vi "calcualte_jv_metrics.vi"(6 "intensity (no. of suns)":string, 9 "Data Array":dbl[][](array[numeric]), 10 "Scan settings":T2={"J-V scan"=TRUE, "Start voltage (V)"=0.0, "End voltage (V)"=0.0, "Step voltage (V)"=1.4, "Scan both directions"=TRUE, "Inverted device structure"=FALSE, "Measurement delay (ms)"=10.0, "Measurement speed"=0, "Scan rate (V/s)"=0.0, "Stabilisation time (s)"=0.0, "Stabilisation mode"=0, "Stabilisation value (V or A) "=1.0, "Illumination"=0, "Stabilisation in the dark?"=FALSE, "Repeat light scans"=FALSE, "No. of repeat scans"=0.0, "Only repeat for best pixel"=1, "J-t scan"=FALSE, "J-t best pixel only"=7, "J-t start voltage (V)"=0.0, "J-t end voltage (V)"=1.4, "J-t step voltage (V)"=0.01, "Step time (s)"=0.7, "J-t scan both directions"=TRUE, "J-t inverted device structure"=FALSE, "Settling delay (s)"=0.0, "J-t measurement speed"=0, "J-t illumination"=2, "Max. power stabilisation"=FALSE, "Max power best pixel only"=1, "Max. power point tracker"=FALSE, "Vmp from J-V scan"=FALSE, "Max P stab. Specific voltage"=FALSE, "Vmp (V)"=1.0, "Stabilisation time step (s)"=1.0, "Total stabilisation time (s)"=100.0} {"Settling delay (s)" min=0.0; "J-t illumination" items=["Light only", "Dark only", "Light then dark", "Dark then light"]; "Measurement speed" items=["Fast", "Normal", "High accuracy"]; "Illumination" items=["Light only", "Dark only", "Light then dark", "Dark then light"]; "Only repeat for best pixel" items=["only for best pixel", "for best 2 pixels", "for best 3 pixels", "for best 4 pixels", "for best 5 pixels", "for best 6 pixels", "for best 7 pixels", "for all pixels"]; "No. of repeat scans" min=1.0 step=1.0; "Max power best pixel only" items=["only the best pixel", "the best 2 pixels", "the best 3 pixels", "the best 4 pixels", "the best 5 pixels", "the best 6 pixels", "the best 7 pixels", "all pixels"]; "J-t best pixel only" items=["only the best pixel", "the best 2 pixels", "the best 3 pixels", "the best 4 pixels", "the best 5 pixels", "the best 6 pixels", "the best 7 pixels", "all pixels"]; "J-t measurement speed" items=["Fast", "Normal", "High Accuracy"]; "Stabilisation mode" items=["V", "I"]; "Measurement delay (ms)" min=10.0}, 11 "Cell details cluster":T1={"Cell Position"=16, "Cell Label"="", "Pixel to measure"=0, "Area (cm^2)"=0.126, "Variable"="", "Variable value"="", "Scan settings in queue"=0, "Light or dark"="", "Measurement type"=""} {"Pixel to measure" items=["All", "1", "2", "3", "4", "5", "6", "7", "8"]}) -> (1 "j-v metrics":string[](array[string]), 2 "j-v data":string[][](array[string]))   [LabVIEW 2016]
uses:
  TypeDefs/scan_settings.ctl
  <vilib>/Analysis/NI_AALPro.lvlib
panel:
  out "Vmp":dbl
  out "PCE":dbl
  out "FF":dbl
  out "Voc":dbl
  out "Jsc":dbl
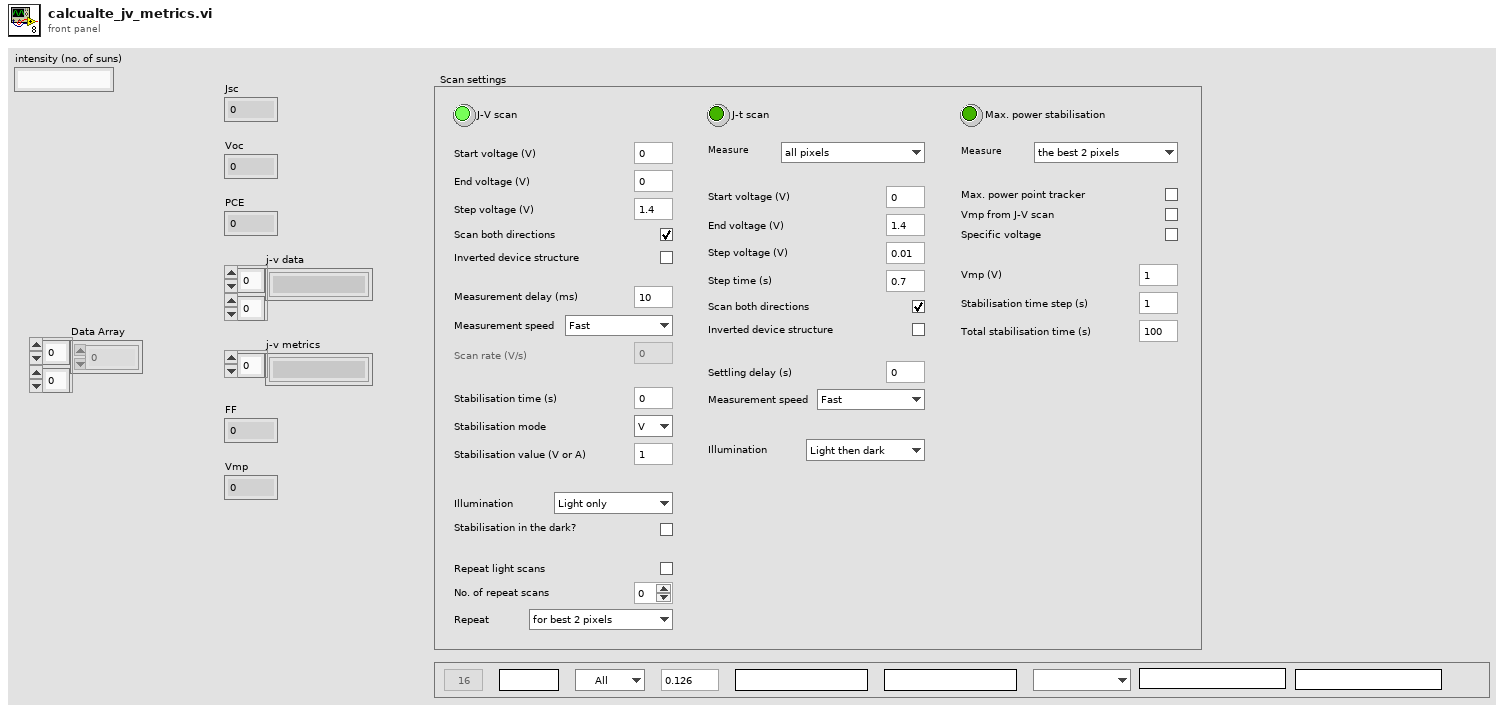
[diagram p1: front panel]
types:
  T1 = cluster{"Cell Position":i32, "Cell Label":string, "Pixel to measure":u16, "Area (cm^2)":dbl, "Variable":string, "Variable value":string, "Scan settings in queue":u16, "Light or dark":string, "Measurement type":string}
  T2 = typedef "scan_settings.ctl" = cluster{"J-V scan":bool, "Start voltage (V)":dbl, "End voltage (V)":dbl, "Step voltage (V)":dbl, "Scan both directions":bool, "Inverted device structure":bool, "Measurement delay (ms)":dbl, "Measurement speed":u8, "Scan rate (V/s)":dbl, "Stabilisation time (s)":dbl, "Stabilisation mode":u16, "Stabilisation value (V or A) ":dbl, "Illumination":u16, "Stabilisation in the dark?":bool, "Repeat light scans":bool, "No. of repeat scans":dbl, "Only repeat for best pixel":u16, "J-t scan":bool, "J-t best pixel only":u16, "J-t start voltage (V)":dbl, "J-t end voltage (V)":dbl, "J-t step voltage (V)":dbl, "Step time (s)":dbl, "J-t scan both directions":bool, "J-t inverted device structure":bool, "Settling delay (s)":dbl, "J-t measurement speed":u16, "J-t illumination":u16, "Max. power stabilisation":bool, "Max power best pixel only":u16, "Max. power point tracker":bool, "Vmp from J-V scan":bool, "Max P stab. Specific voltage":bool, "Vmp (V)":dbl, "Stabilisation time step (s)":dbl, "Total stabilisation time (s)":dbl}
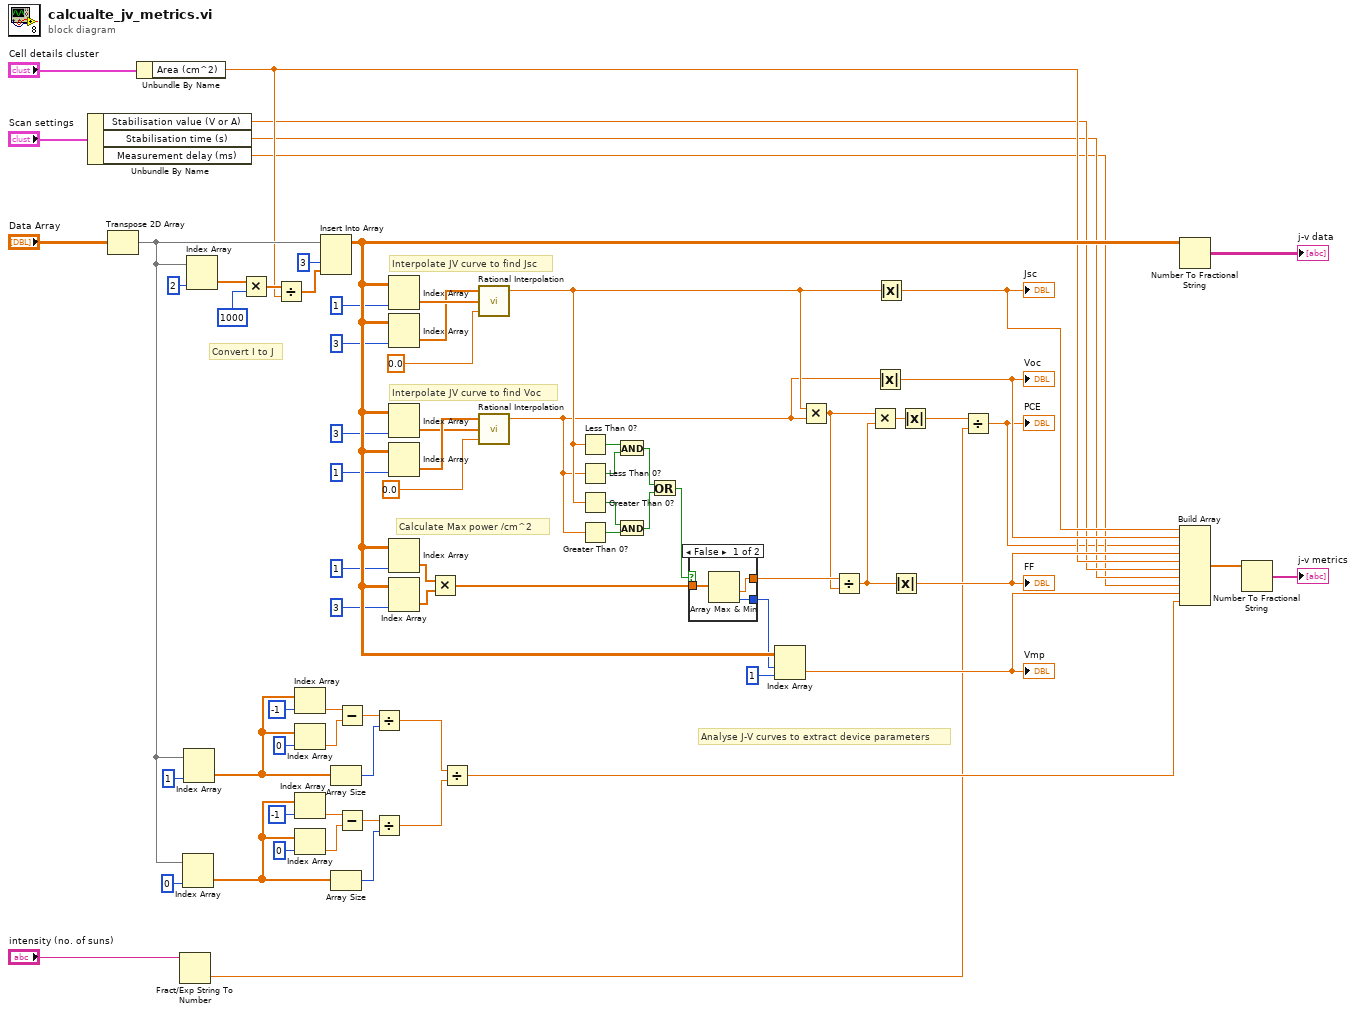
[diagram p0: block diagram]
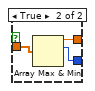
[diagram p2: hidden frame]
diagram:
  # "Convert I to J"
  # "Calculate Max power /cm^2"
  # "Interpolate JV curve to find Voc"
  # "Interpolate JV curve to find Jsc"
  # "Analyse J-V curves to extract device parameters"
  n1 = Unbundle By Name("Scan settings") -> ("Stabilisation value (V or A)"=w7:dbl, "Stabilisation time (s)"=w6:dbl, "Measurement delay (ms)"=w5:dbl)
  n2 = Transpose 2D Array(2D array="Data Array") -> (transposed array=w55:dbl[][])
  n3 = Unbundle By Name("Cell details cluster") -> ("Area (cm^2)"=w9:dbl)
  n4 = Fract/Exp String To Number(string="intensity (no. of suns)") -> (number=w1:dbl)  [unwired: 3 in, 1 out]
  n5 = Index Array(array=w55, index (col)=0 ("disabled index (col)")) -> (element=w62:dbl[])  [unwired: 1 in]
  n6 = Index Array(array=w55, index (col)=1 ("disabled index (col)")) -> (element=w71:dbl[])  [unwired: 1 in]
  n7 = Index Array(array=w55, index (col)=2) -> (element=w45:dbl[])  [unwired: 1 in]
  n8 = Multiply(x=w45, y=1000) -> (x*y=w47:dbl[])
  n9 = Divide(x=w47, y=w9) -> (x/y=w48:dbl[])
  n10 = Index Array(array=w71, index=-1) -> (element=w67:dbl)
  n11 = Index Array(array=w71, index=0) -> (element=w68:dbl)
  n12 = Index Array(array=w62, index=-1) -> (element=w60:dbl)
  n13 = Index Array(array=w62, index=0) -> (element=w61:dbl)
  n14 = Insert Into Array(array=w55, index (col)=3, new element=w48) -> (w52:dbl[][])  [unwired: 1 in]
  n15 = Array Size(array=w71) -> (size(s)=w70:i32)
  n16 = Array Size(array=w62) -> (size(s)=w64:i32)
  n17 = Subtract(x=w67, y=w68) -> (x-y=w69:dbl)
  n18 = Subtract(x=w60, y=w61) -> (x-y=w63:dbl)
  n19 = Divide(x=w69, y=w70) -> (x/y=w72:dbl)
  n20 = Divide(x=w63, y=w64) -> (x/y=w73:dbl)
  n21 = Index Array(array=w52, index (col)=1) -> (element=w22:dbl[])  [unwired: 1 in]
  n22 = Index Array(array=w52, index (col)=3) -> (element=w21:dbl[])  [unwired: 1 in]
  n23 = Index Array(array=w52, index (col)=3) -> (element=w23:dbl[])  [unwired: 1 in]
  n24 = Index Array(array=w52, index (col)=1) -> (element=w25:dbl[])  [unwired: 1 in]
  n25 = Index Array(array=w52, index (col)=1) -> (element=w17:dbl[])  [unwired: 1 in]
  n26 = Index Array(array=w52, index (col)=3) -> (element=w18:dbl[])  [unwired: 1 in]
  n27 = Multiply(x=w17, y=w18) -> (x*y=w24:dbl[])
  n28 = Divide(x=w72, y=w73) -> (x/y=w74:dbl)
  n29 = call <vilib>:"Rational Interpolation.vi"("x value"=0.0, "X"=w22, "Y"=w21) -> ("interpolation value"=w46:dbl)  [unwired: 2 out]
  n30 = call <vilib>:"Rational Interpolation.vi"("x value"=0.0, "X"=w23, "Y"=w25) -> ("interpolation value"=w38:dbl)  [unwired: 2 out]
  n31 = Less Than 0?(x=w46) -> (x < 0?=w32:bool)
  n32 = Less Than 0?(x=w38) -> (x < 0?=w35:bool)
  n33 = Greater Than 0?(x=w46) -> (x > 0?=w34:bool)
  n34 = Greater Than 0?(x=w38) -> (x > 0?=w33:bool)
  n35 = And(x=w32, y=w35) -> (x .and. y?=w30:bool)
  n36 = And(x=w34, y=w33) -> (x .and. y?=w31:bool)
  n37 = Or(x=w30, y=w31) -> (x .or. y?=w36:bool)
  n38 = case shown="False" w36 {
    tunnel: [w77 w81] -> w49
    tunnel: w24 -> [w78 w80]
    tunnel: [w76 w79] -> w51
    frame False {
      n39 = Array Max & Min(array=w78) -> (min value=w77:dbl, min index (indices)=w76:i32)  [unwired: 2 out]
    }
    frame True {
      n40 = Array Max & Min(array=w80) -> (max value=w81:dbl, max index (indices)=w79:i32)  [unwired: 2 out]
    }
  }
  n41 = Index Array(array=w52, index (row)=w51, index (col)=1) -> (element=w53:dbl)
  "Vmp" <- w53
  n42 = Multiply(x=w46, y=w38) -> (x*y=w26:dbl)
  n43 = Divide(x=w49, y=w26) -> (x/y=w41:dbl)
  n44 = Multiply(x=w26, y=w41) -> (x*y=w40:dbl)
  n45 = Absolute Value(x=w38) -> (abs(x)=w39:dbl)
  "Voc" <- w39
  n46 = Absolute Value(x=w46) -> (abs(x)=w37:dbl)
  "Jsc" <- w37
  n47 = Absolute Value(x=w41) -> (abs(x)=w42:dbl)
  "FF" <- w42
  n48 = Absolute Value(x=w40) -> (abs(x)=w3:dbl)
  n49 = Divide(x=w3, y=w1) -> (x/y=w2:dbl)
  "PCE" <- w2
  n50 = Number To Fractional String(number=w52) -> (F-format string=→"j-v data":string[][])  [unwired: 3 in]
  n51 = Build Array(w37, w39, w2, w42, w9, w7, w6, w5, w53, w74) -> (w27:dbl[])
  n52 = Number To Fractional String(number=w27) -> (F-format string=→"j-v metrics":string[])  [unwired: 3 in]
